vi "Concatenate_Blocks.vi"() -> (5 "Plug in titles":string[](array[string]), 7 "Plug in values":string[](array[string]))   [LabVIEW 2012]
uses:
  <vilib>/Analysis/2dsp.llb/Integral Method.ctl
  Controls/Post_Process.ctl
  Controls/Graph_Type.ctl
  Globals/Meas_global.vi
  <vilib>/Analysis/8numeric.llb/1D Numeric Integration.vi
  <vilib>/Analysis/NI_AALBase.lvlib
  <vilib>/Analysis/NI_AALPro.lvlib
panel:
  out "Integral (u^2)":dbl format="%0.4f"
  in  "integration method":T1 items=["Trapezoidal Rule", "Simpson's Rule", "Simpson's 3/8 Rule", "Bode Rule"]
  in  "PDF":bool=TRUE
  out "No Of Spectral Averages":i32
  out "Autocorrelation":cluster{dbl, dbl, dbl[]}[](graph)
  in  "Show Smooth":bool=TRUE
  in  "Save Plots":bool
  in  "No of averged samples in spectra":i32=4096
  in  "Calculate Spectra and Histogram?":bool
  out "Spectra":cluster{dbl, dbl, dbl[]}[](graph)
  in  "Averaging samples":i32=5 min=1 max=1000
  out "Histogram/Pdf":T2(graph)
  out "Waveform Graph":dbl[][](graph)
  in  "Channels to Plot":i32[](array[ring])=[0] items=["Pitot (URef)", "Mano (5HP1)", "Mano (5HP2)", "Mano (5HP3)", "Mano (5HP4)", "Mano (5HP5)", "HW (Uhf)", "Save Nothing"]
  # "Run this VI to update the channel names"
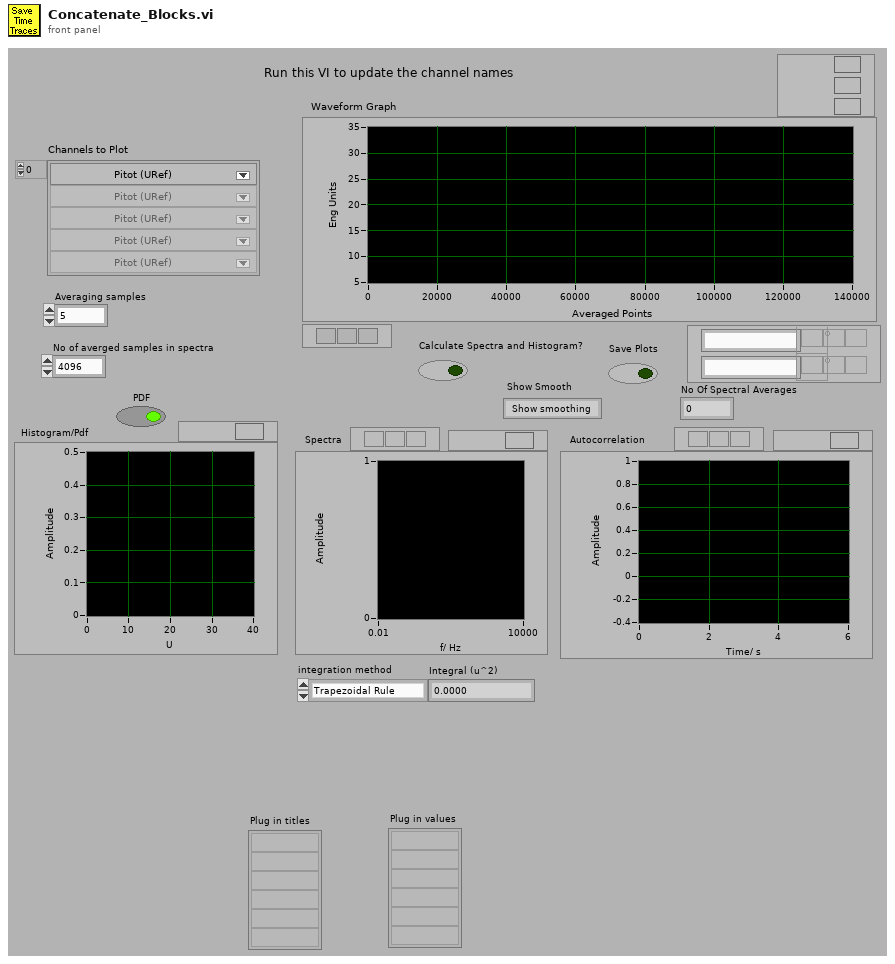
[diagram p1: front panel]
types:
  T1 = typedef "NI_AALPro.lvlib/Integral Method.ctl" = i32
  T2 = cluster{"element":dbl, dbl, "1D histogram or PDF":dbl[]}[]
  T3 = typedef "Analysis_info_cluster.ctl" = cluster{"Colour":u32, "Inst type":T4, "Inst name":string, "Symbol":string, "Code name":string, "Extra Info":string, "Inst Array":T5, "Extra Titles":string[], "Extra Values":string[], "U":dbl, "u^2":dbl, "u^3":dbl, "u^4":dbl, "Skew_u":dbl, "Kurt_u":dbl, "Sd Error in Mean":dbl, "% u'/U":dbl, "X":dbl, "Y":dbl, "Z":dbl, "Timescale integral to 25%":dbl, "Sd Error in Variance":dbl, "Calib File":path, "Calib Constants":dbl[], "Output Position":bool, "Full Stats":bool, "Av Sampling Rate":dbl, "Av No of Samples":dbl, "Total Meas Time (s)":dbl, "ADAM Ch Name":string}
  T4 = typedef "Inst_type.ctl" = enum16{"Propeller anemometer", "Raw voltage", "Pressure Transducer", "Pitot-static tube", "Preston tube", "Hot wire", "Cross wire 1", "Cross wire 2", "Generic Linear", "Generic Polynomial", "Generic BackPoly", "Fast FID", "Thermocouple", "Cold wire", "Pulsed Wire", "LDA Vel", "LDA Tran time", "LDA Arr time"}
  T5 = typedef "Instrument_Array.ctl" = enum16{"PWA", "LDA", "Analogue"}
  T6 = typedef "Time_Trace_Cluster.ctl" = cluster{"Weighting":dbl[], "Time (s)":dbl[], "Voltage":dbl[], "Eng Values":dbl[]}
  T7 = typedef "Post_Process.ctl" = enum16{"Take New Data", "Post Process Raw Data File"}
  T8 = typedef "Graph_Type.ctl" = enum16{"Show no graph", "Voltage trace", "Velocity trace", "Vel histogram", "Spectrum", "f.E(f) v Log f", "Auto-Corr"}
  T9 = cluster{"Plot 1":u16, "Plot 2":u16, "Save graph":u16, "Plot Type":T8}
  T10 = cluster{"element":dbl, dbl, "1D histogram or PDF":dbl[]}
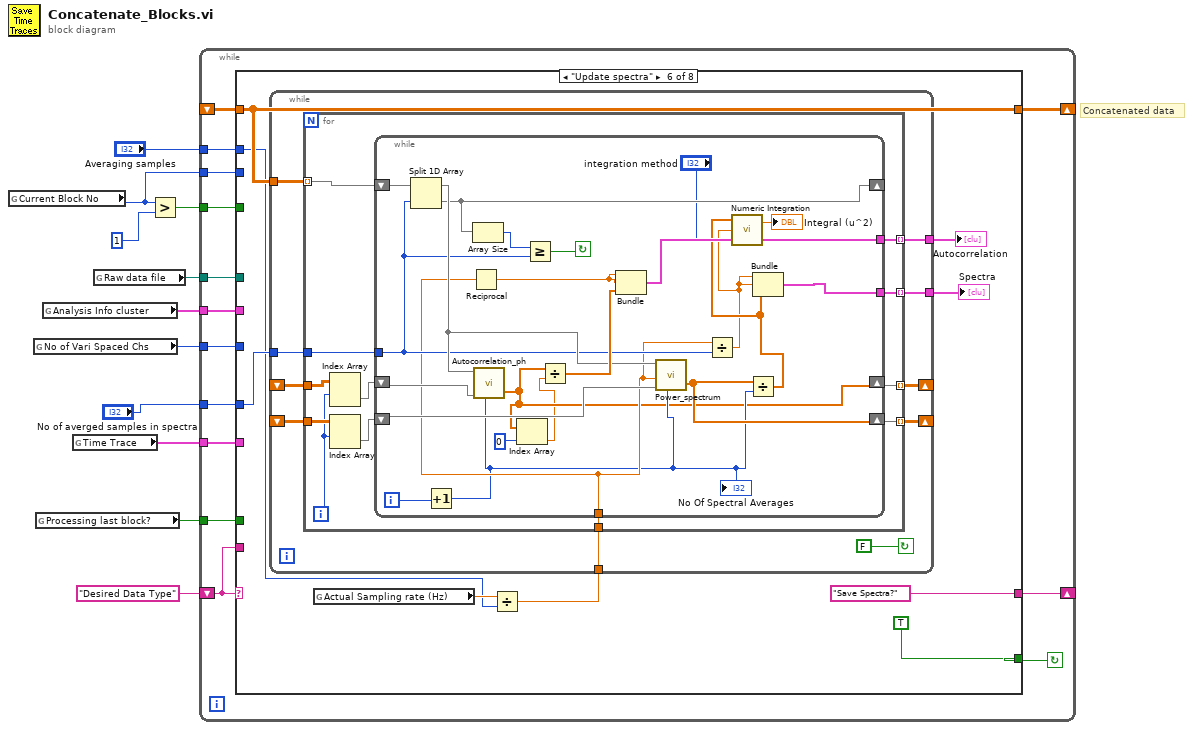
[diagram p0: block diagram]
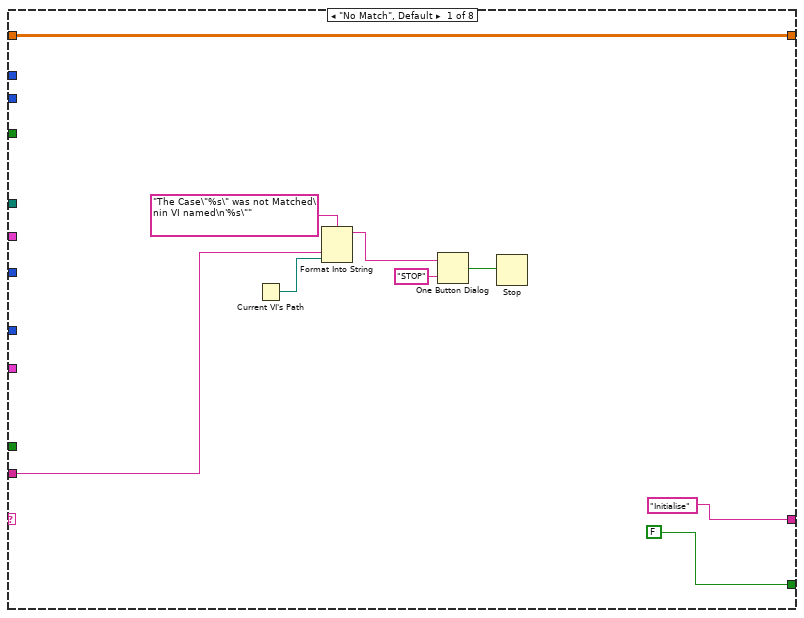
[diagram p2: hidden frame]
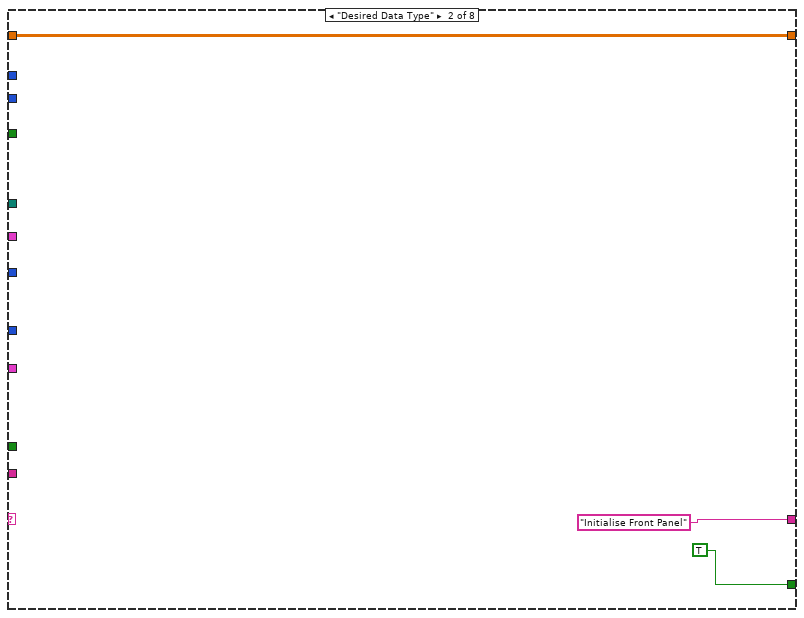
[diagram p3: hidden frame]
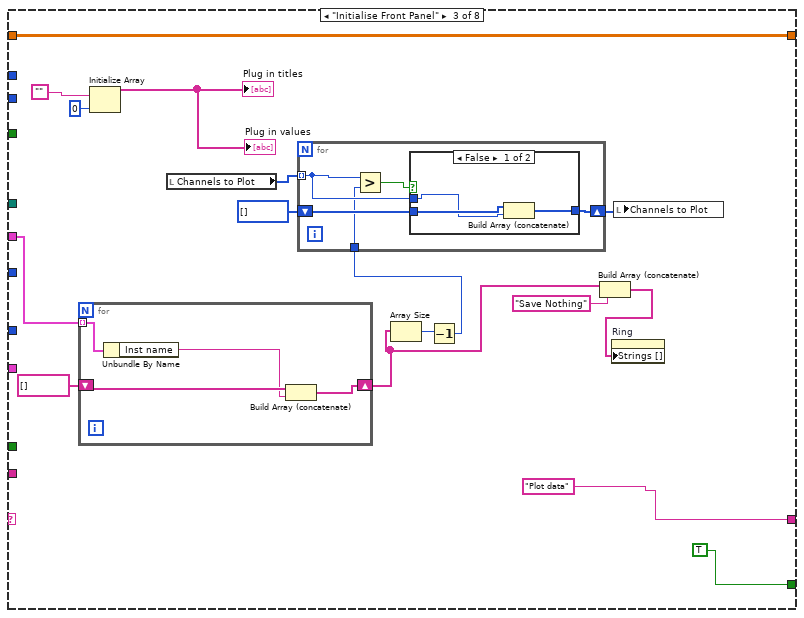
[diagram p4: hidden frame]
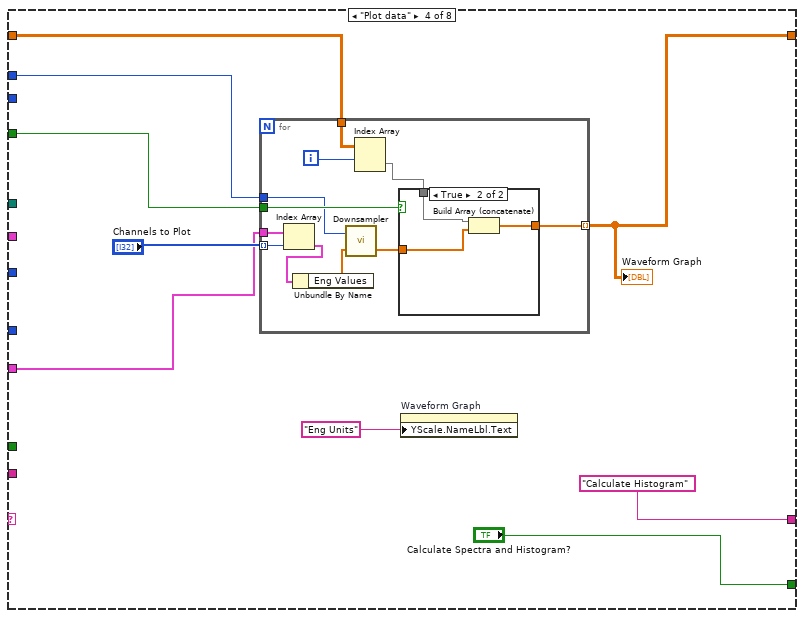
[diagram p6: hidden frame]
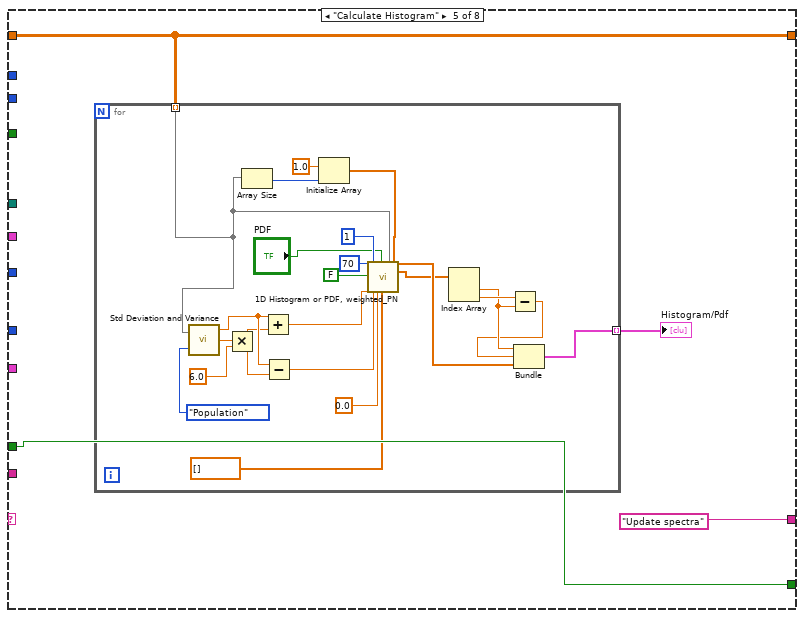
[diagram p8: hidden frame]
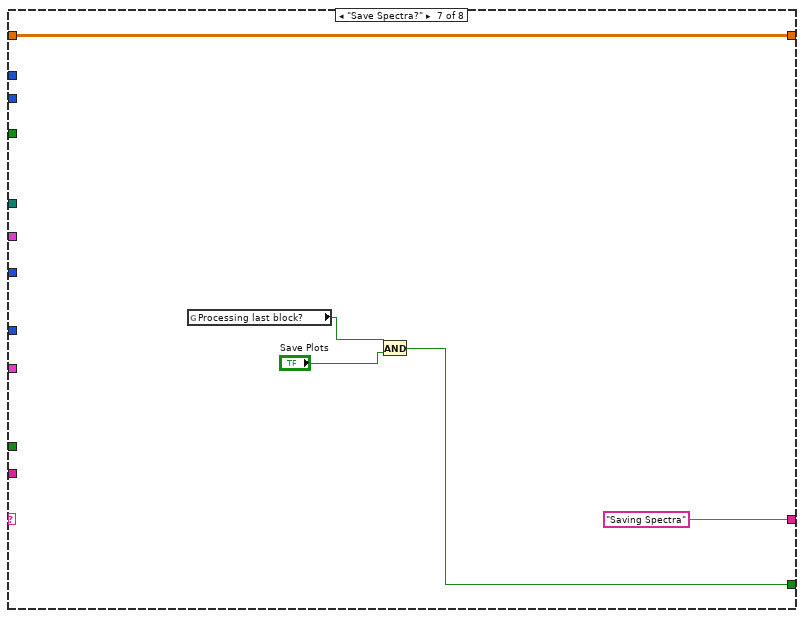
[diagram p9: hidden frame]
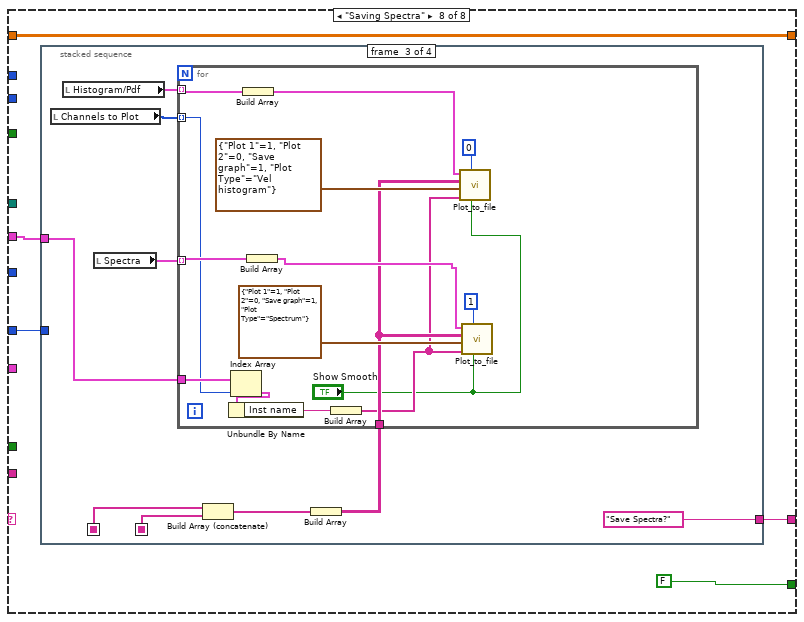
[diagram p10: hidden frame]
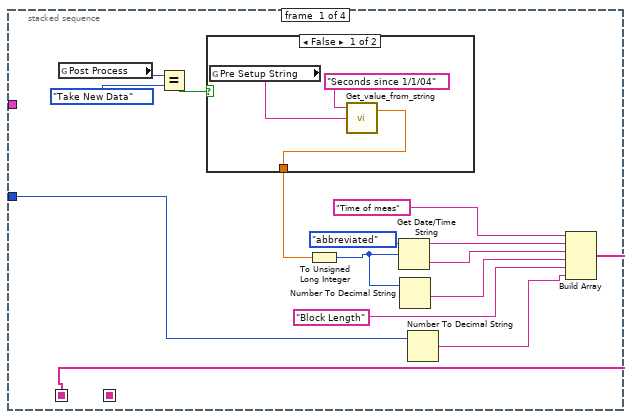
[diagram p11: hidden frame]
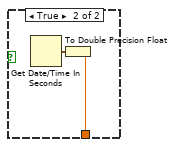
[diagram p12: hidden frame]
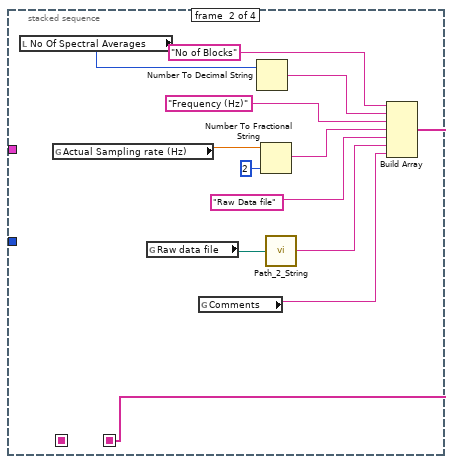
[diagram p13: hidden frame]
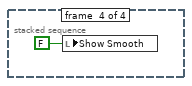
[diagram p14: hidden frame]
diagram:
  # "Concatenated data"
  n1 = global read "Meas_global.vi" "Current Block No"() -> (w8:i32)
  n2 = global read "Meas_global.vi" "No of Vari Spaced Chs"() -> (w6:i32)
  n3 = global read "Meas_global.vi" "Processing last block?"() -> (w1:bool)
  n4 = global read "Meas_global.vi" "Analysis Info cluster"() -> (w7:T3[])
  n5 = global read "Meas_global.vi" "Time Trace"() -> (w3:T6[])
  n6 = global read "Meas_global.vi" "Raw data file"() -> (w10:path)
  n7 = Greater?(x=w8, y=1) -> (0:w5:bool)
  n8 = while {
    shift-left: "Desired Data Type" -> [w23]
    shift-right: [w24] -> _
    tunnel: w10 -> [w22]
    tunnel: w5 -> [w21]
    tunnel: w8 -> [w20]
    tunnel: w7 -> [w19]
    tunnel: w6 -> [w18]
    shift-right: [w16] -> _
    shift-left: _ -> [w17]
    tunnel: "No of averged samples in spectra" -> [w15]
    tunnel: w3 -> [w14]
    tunnel: "Averaging samples" -> [w13]
    tunnel: w1 -> [w12]
    stop <- w25 continue-if-true
    n9 = case shown="\"Update spectra\"" w23 {
      tunnel: [FALSE TRUE TRUE "Calculate Spectra and Histogram?" w92 TRUE ("Calculate Spectra and Histogram?") w172 FALSE ("Calculate Spectra and Histogram?")] -> w25
      tunnel: ["Initialise" "Initialise Front Panel" "Plot data" "Calculate Histogram" ("t") "Update spectra" "Save Spectra?" "Saving Spectra" w180] -> w24
      tunnel: w23 -> [w29 _ _ _ _ _ _ _]
      tunnel: w22 -> [_ _ _ _ _ _ _ _]
      tunnel: w21 -> [_ _ _ w74 _ _ _ _]
      tunnel: w20 -> [_ _ _ _ _ _ _ _]
      tunnel: w19 -> [_ _ w40 _ _ _ _ w179]
      tunnel: w18 -> [_ _ _ _ _ _ _ _]
      tunnel: w17 -> [w26 w35 w43 w75 w94 w123 w176 w181]
      tunnel: [w26 w35 w43 w72 w94 w123 w176 w181] -> w16
      tunnel: w15 -> [_ _ _ _ _ w124 _ w177]
      tunnel: w14 -> [_ _ _ w68 _ _ _ _]
      tunnel: w13 -> [_ _ _ w67 _ w121 _ _]
      tunnel: w12 -> [_ _ _ _ w92 _ _ _]
      frame "No Match", Default {
        n10 = Current VI's Path() -> (path=w28:path)
        n11 = Format Into String(format string="The Case\"%s\" was not Matched\nin VI named\n'%s\"" ("Format String"), w29, w28) -> (resulting string=w32:string)  [unwired: 2 in, 1 out]
        n12 = One Button Dialog(message=w32, button name ("OK")="STOP") -> (true=w30:bool)
        n13 = Stop(stop? (T)=w30) -> ()
      }
      frame "Desired Data Type" {
      }
      frame "Initialise Front Panel" {
        n14 = for {
          tunnel: w40 -> [w57] mode=indexing
          shift-right: [w55] -> w39
          shift-left: string[] [] -> [w56]
          n15 = Unbundle By Name(w57) -> ("Inst name"=w54:string)
          n16 = Build Array (concatenate)(w56, w54) -> (w55:string[])
        }
        n17 = Initialize Array("", 0) -> (→"Plug in values" →"Plug in titles":string[])
        n18 = local read "Channels to Plot"() -> (w50:i32[])
        n19 = Array Size(array=w39) -> (size(s)=w45:i32)
        n20 = Decrement(x=w45) -> (x-1=w44:i32)
        n21 = for {
          tunnel: w50 -> [w59] mode=indexing
          shift-right: [w60] -> w48
          shift-left: i32[] [] -> [w61]
          tunnel: w44 -> [w58]
          n22 = Greater?(x=w59, y=w58) -> (0:w62:bool)
          n23 = case shown="False" w62 {
            tunnel: w61 -> [w65 w66]
            tunnel: [w64 w66] -> w60
            tunnel: w59 -> [w63 _]
            frame False {
              n24 = Build Array (concatenate)(w65, w63) -> (w64:i32[])
            }
            frame True {
            }
          }
        }
        n25 = Build Array (concatenate)(w39, "Save Nothing") -> (w46:string[])
        n26 = property on="Ring" class="Ring (strict)"("Strings []"=w46) -> ()  [unwired: 2 in, 2 out]
        n27 = local write "Channels to Plot"(w48) -> ()
      }
      frame "Plot data" {
        n28 = for {
          tunnel: w68 -> [w86]
          tunnel: "Channels to Plot" -> [w85] mode=indexing
          tunnel: w75 -> [w82]
          tunnel: [w83] -> w72 mode=indexing
          tunnel: w74 -> [w84]
          tunnel: w67 -> [w76]
          i -> [w81]
          n29 = Index Array(array=w86, index=w85) -> (element=w78:T6)
          n30 = Unbundle By Name(w78) -> ("Eng Values"=w77:dbl[])
          n31 = call "Downsampler.vi"("Input Array"=w77, "Averaging samples"=w76) -> ("Downsampled Array"=w79:dbl[])  [unwired: 1 out]
          n32 = Index Array(array=w82, index (row)=w81) -> (element=w80:dbl[])  [unwired: 1 in]
          n33 = case shown="True" w84 {
            tunnel: w80 -> [_ w90]
            tunnel: w79 -> [w87 w89]
            tunnel: [w87 w88] -> w83
            frame False {
            }
            frame True {
              n34 = Build Array (concatenate)(w90, w89) -> (w88:dbl[])
            }
          }
        }
        "Waveform Graph" <- w72
        n35 = property on="Waveform Graph" class="WFGraph (strict)"("YScale.NameLbl.Text"="Eng Units") -> ()  [unwired: 2 in, 2 out]
      }
      frame "Calculate Histogram" {
        n36 = for {
          tunnel: w94 -> [w95] mode=indexing
          tunnel: [w96] -> w91 mode=indexing
          n37 = call <vilib>:"Std Deviation and Variance.vi"("X"=w95, "Weighting (Sample)"=enum16{"Sample", "Population"}."Population") -> ("mean"=w110:dbl, "standard deviation"=w109:dbl)  [unwired: 1 out]
          n38 = Multiply(x=w109, y=6.0) -> (x*y=w107:dbl)
          n39 = Array Size(array=w95) -> (size(s)=w114:i32)
          n40 = Add(x=w110, y=w107) -> (x+y=w105:dbl)
          n41 = Subtract(x=w110, y=w107) -> (x-y=w104:dbl)
          n42 = Initialize Array(1.0 ("element"), w114) -> (w112:dbl[])
          n43 = call "1D Histogram or PDF, weighted_PN.vi"("Nbins"=70, "Mean shift"=FALSE, "max"=w105, "Current block no."=1, "min"=w104, "Shift SumW in"=0.0, "PDF"="PDF", "Shift PDF in"=dbl[] [], "1D data"=w95, "Weights"=w112) -> ("1D histogram or PDF"=w111:dbl[], "bin centre vals."=w100:dbl[])  [unwired: 13 in, 3 out]
          n44 = Index Array(array=w100) -> (element #1=w98:dbl, element #2=w99:dbl)  [unwired: 2 in]
          n45 = Subtract(x=w99, y=w98) -> (x-y=w97:dbl)
          n46 = Bundle("element"=w98, w97, "1D histogram or PDF"=w111) -> (w96:T10)  [unwired: 1 out]
        }
        "Histogram/Pdf" <- w91
      }
      frame "Update spectra" {
        n47 = global read "Meas_global.vi" "Actual Sampling rate (Hz)"() -> (w122:dbl)
        n48 = Divide(x=w122, y=w121) -> (x/y=w120:dbl)
        n49 = while {
          shift-left: _ -> [w133]
          shift-right: [w136] -> _
          tunnel: w124 -> [w134]
          shift-right: [w131] -> _
          shift-left: _ -> [w132]
          tunnel: w123 -> [w130]
          tunnel: w120 -> [w129]
          tunnel: [w128] -> w119
          tunnel: [w127] -> w118
          stop <- FALSE continue-if-true
          n50 = for {
            tunnel: [w145] -> w136 mode=indexing
            tunnel: w134 -> [w148]
            tunnel: w133 -> [w141]
            tunnel: w132 -> [w143]
            tunnel: [w146] -> w131 mode=indexing
            tunnel: w130 -> [w147] mode=indexing
            tunnel: w129 -> [w144]
            tunnel: [w138] -> w128 mode=indexing
            tunnel: [w137] -> w127 mode=indexing
            i -> [w139]
            n51 = Index Array(array=w143, index (row)=w139) -> (element=w142:dbl[])  [unwired: 1 in]
            n52 = Index Array(array=w141, index (row)=w139) -> (element=w140:dbl[])  [unwired: 1 in]
            n53 = while {
              tunnel: w148 -> [w164]
              shift-right: [w158] -> _
              shift-left: w147 -> [w161]
              shift-right: [w169] -> w145
              shift-left: w140 -> [w167]
              shift-right: [w154] -> w146
              shift-left: w142 -> [w168]
              tunnel: w144 -> [w162]
              tunnel: [w160] -> w138
              tunnel: [w159] -> w137
              i -> [w157]
              stop <- w163 continue-if-true
              n54 = Split 1D Array(array=w161, index=w164) -> (first subarray=w166:dbl[], second subarray=w158:dbl[])
              n55 = Increment(x=w157) -> (x+1=w156:i32)
              "No Of Spectral Averages" <- w156
              n56 = Reciprocal(x=w162) -> (1/x=w171:dbl)
              n57 = Array Size(array=w158) -> (size(s)=w165:i32)
              n58 = call "Autocorrelation_ph.vi"("X"=w166, "Autocorrelation of X"=w168, "Block No"=w156) -> ("Autocorrelation of X"=w154:dbl[])  [unwired: 3 in]
              n59 = Index Array(array=w154, index=0 ("Index")) -> (element=w153:dbl)
              n60 = Greater Or Equal?(x=w165, y=w164) -> (x >= y?=w163:bool)
              n61 = Divide(x=w154, y=w153) -> (x/y=w170:dbl[])
              n62 = Bundle(w171, w171, w170) -> (w160:cluster{dbl, dbl, dbl[]})  [unwired: 1 out]
              n63 = call "Power_spectrum.vi"("U"=w166, "Sampling frequency"=w162, "Spectrum input array"=w167, "Block No"=w156) -> ("Spectrum output array"=w169:dbl[])  [unwired: 1 in, 1 out]
              n64 = Divide(x=w162, y=w164) -> (x/y=w149:dbl)
              n65 = Divide(x=w169, y=w156) -> (x/y=w150:dbl[])
              n66 = call-poly <vilib>:"Numeric Integration.vi"("integration method"="integration method", "dt"=w149, "Input Array"=w150) -> ("result"=→"Integral (u^2)":dbl)  [unwired: 1 out]
              n67 = Bundle(w149, w149, w150) -> (w159:cluster{dbl, dbl, dbl[]})  [unwired: 1 out]
            }
          }
        }
        "Spectra" <- w118
        "Autocorrelation" <- w119
      }
      frame "Save Spectra?" {
        n68 = global read "Meas_global.vi" "Processing last block?"() -> (w173:bool)
        n69 = And(x=w173, y="Save Plots") -> (x .and. y?=w172:bool)
      }
      frame "Saving Spectra" {
        n70 = stacked-sequence {
          seq-local: [w185 _ _ _] -> [_ _ w220 _]
          seq-local: [_ w204 _ _] -> [_ _ w219 _]
          tunnel: [_ _ "Save Spectra?" _] -> w180
          tunnel: w179 -> [_ _ w214 _]
          tunnel: w177 -> [w183 _ _ _]
          frame #0 {
            n71 = global read "Meas_global.vi" "Post Process"() -> (w187:T7)
            n72 = Equal?(x=w187, y=Post_Process."Take New Data" ("Post Process")) -> (x = y?=w188:bool)
            n73 = case shown="False" w188 {
              tunnel: [w196 w200] -> w189
              frame False {
                n74 = global read "Meas_global.vi" "Pre Setup String"() -> (w197:string)
                n75 = call "Get_value_from_string.vi"("Input string"=w197, "Variable name"="Seconds since 1/1/04") -> ("Value"=w196:dbl)  [unwired: 1 in, 1 out]
              }
              frame True {
                n76 = Get Date/Time In Seconds() -> (seconds since 1Jan1904=w199:timestamp)
                n77 = To Double Precision Float(number=w199) -> (double precision float=w200:dbl)
              }
            }
            n78 = To Unsigned Long Integer(number=w189) -> (unsigned 32bit integer=w193:u32)
            n79 = Get Date/Time String(date format (0)=enum16{"short", "long", "abbreviated"}."abbreviated", seconds (now)=w193) -> (date string=w191:string, time string=w192:string)  [unwired: 1 out]
            n80 = Number To Decimal String(number=w193) -> (decimal integer string=w194:string)  [unwired: 1 out]
            n81 = Number To Decimal String(number=w183) -> (decimal integer string=w182:string)  [unwired: 1 out]
            n82 = Build Array("Time of meas", w191, w192, w194, "Block Length" ("element"), w182) -> (w185:string[])
          }
          frame #1 {
            n83 = local read "No Of Spectral Averages"() -> (w201:i32)
            n84 = global read "Meas_global.vi" "Actual Sampling rate (Hz)"() -> (w205:dbl)
            n85 = global read "Meas_global.vi" "Raw data file"() -> (w211:path)
            n86 = global read "Meas_global.vi" "Comments"() -> (w210:string)
            n87 = Number To Decimal String(number=w201) -> (decimal integer string=w202:string)  [unwired: 1 out]
            n88 = Number To Fractional String(number=w205, precision (6)=i16 2) -> (F-format string=w208:string)  [unwired: 2 out]
            n89 = call "Path_2_String.vi"("Real Path"=w211) -> ("Path String"=w212:string)
            n90 = Build Array("No of Blocks", w202, "Frequency (Hz)", w208, "Raw Data file", w212, w210) -> (w204:string[])
          }
          frame #2 {
            n91 = local read "Channels to Plot"() -> (w213:i32[])
            n92 = local read "Histogram/Pdf"() -> (w215:T2)
            n93 = local read "Spectra"() -> (w216:cluster{dbl, dbl, dbl[]}[])
            n94 = Build Array (concatenate)(w220, w219) -> (w218:string[])
            n95 = Build Array(w218) -> (w217:string[][])
            n96 = for {
              tunnel: w217 -> [w225]
              tunnel: w216 -> [w231] mode=indexing
              tunnel: w215 -> [w233] mode=indexing
              tunnel: w214 -> [w229]
              tunnel: w213 -> [w228] mode=indexing
              n97 = Index Array(array=w229, index=w228) -> (element=w226:T3)
              n98 = Unbundle By Name(w226) -> ("Inst name"=w227:string)
              n99 = Build Array(w233) -> (w232:T2)
              n100 = Build Array(w231) -> (w230:cluster{dbl, dbl, dbl[]}[])
              n101 = Build Array(w227) -> (w224:string[])
              n102 = call "Plot_to_file.vi"("Show Smooth"="Show Smooth", "Start trace No"=0, "Trace names"=w224, "Graph"=T9 {"Plot 1"=1, "Plot 2"=0, "Save graph"=1, "Plot Type"=enum."Vel histogram"}, "Plot file label"=w225, "Plot data"=w232) -> ()  [unwired: 6 out]
              n103 = call "Plot_to_file.vi"("Show Smooth"="Show Smooth", "Start trace No"=1, "Trace names"=w224, "Graph"=T9 {"Plot 1"=1, "Plot 2"=0, "Save graph"=1, "Plot Type"=enum."Spectrum"}, "Plot file label"=w225, "Plot data"=w230) -> ()  [unwired: 6 out]
            }
          }
          frame #3 {
            n104 = local write "Show Smooth"(FALSE ("Show Smooth")) -> ()
          }
        }
      }
    }
  }
